vi "ThemalImaging(VDAQ).vi"() -> ()   [LabVIEW 2011]
uses:
  <vilib>/Analysis/1siggen.llb/Riffle Array (I32).vi
  <vilib>/Analysis/NI_AALBase.lvlib
panel:
  in  "选项卡控件":enum32{"前面板", "参数设置"}(tab)
  out "Stim_ID":i32(listbox)=1
  in  "窗口":bool=TRUE
  in  "暂停":bool
  in  "停止":bool
  in  "FramesPerStim":i32=100
  in  "Blk目录":path=path "C:/Documents and Settings/Administrator/桌面/热成像/testblk"
  in  "文件名":string="G4"
  in  "TimeForPrepare(ms)":u32=4000
  in  "InterTrailID":u8
  in  "stim ID":u8[](array[numeric])=[0, 1, 2, 3, 4, 5, 6, 7, 8]
  in  "blk数量":i32=500
  out "错误输出 2":errorcluster
  out "重排的 Stim ID":i32[](array[numeric]) caption="重排的{X}"
  out "重排的 Stim ID Index":i32[](array[numeric]) caption="重排的索引"
  in  "FrameWidth":i32=704
  in  "FrameHeight":i32=576
  in  "Stimuli":i32=5
  out "错误输出":errorcluster
  out "DeInitDSPs":i32
  in  "Brightness":i32(slide) min=0 max=255 scale=0.0..255.0
  in  "Contrast":i32(slide) min=0 max=127 scale=0.0..127.0
  # "开始前一定要改名字"
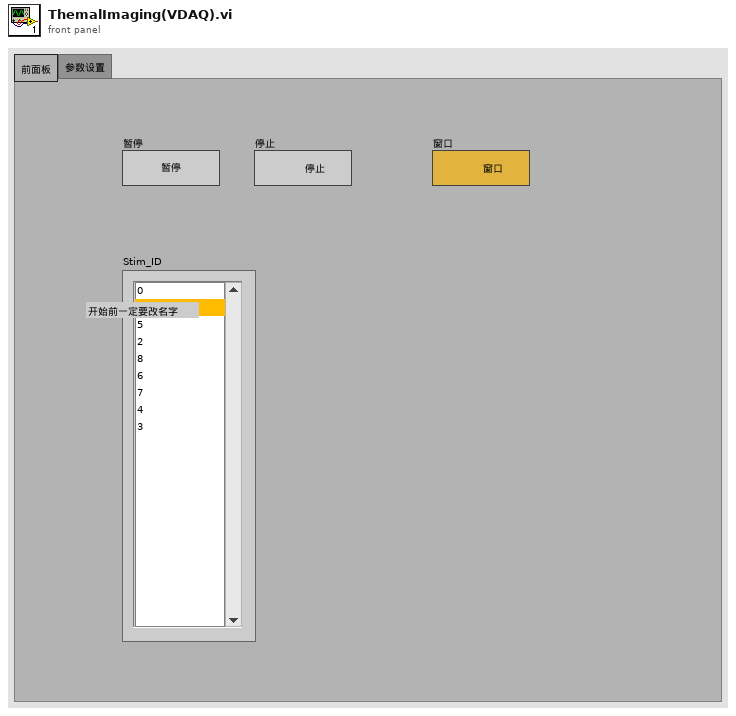
[diagram p1: front panel]
types:
  T1 = typedef "Image Type" = u32
  T2 = typedef "IMAQ Image.ctl" = refnum<image>
  T3 = enum16{"big-endian, network order", "native, host order", "little-endian"}
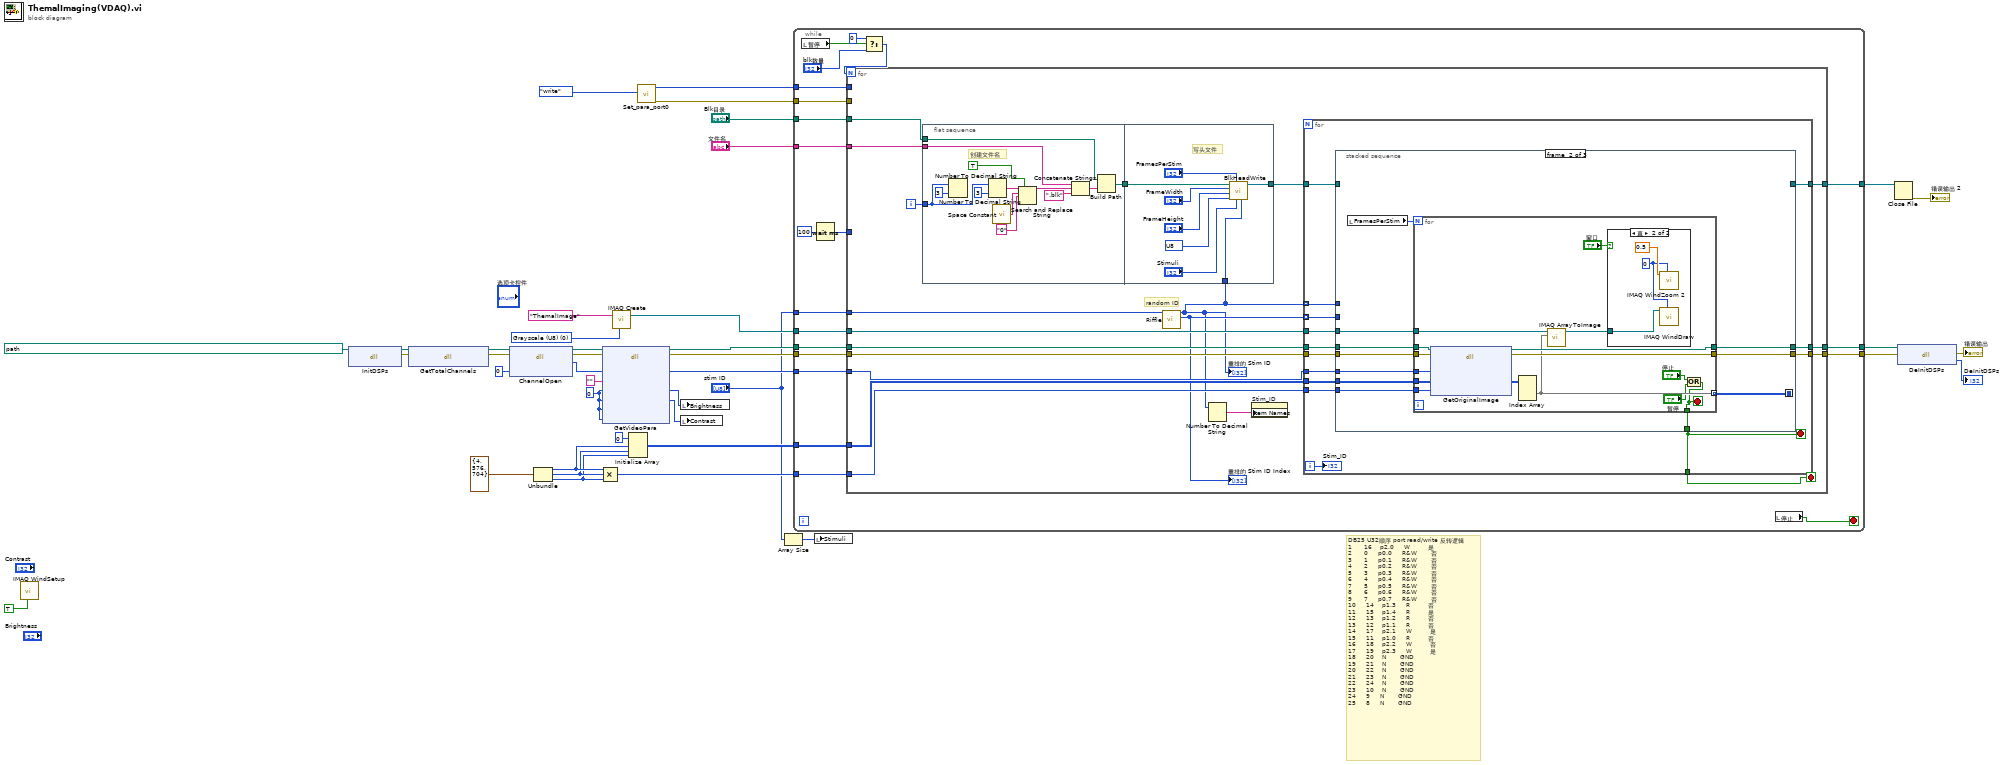
[diagram p0: block diagram]
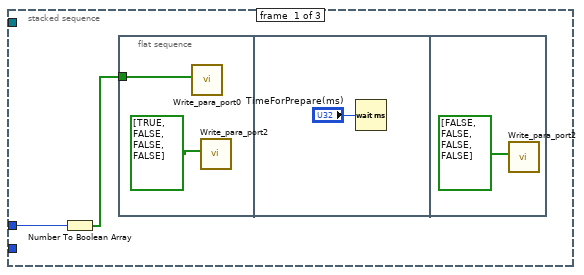
[diagram p2: hidden frame]
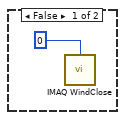
[diagram p3: hidden frame]
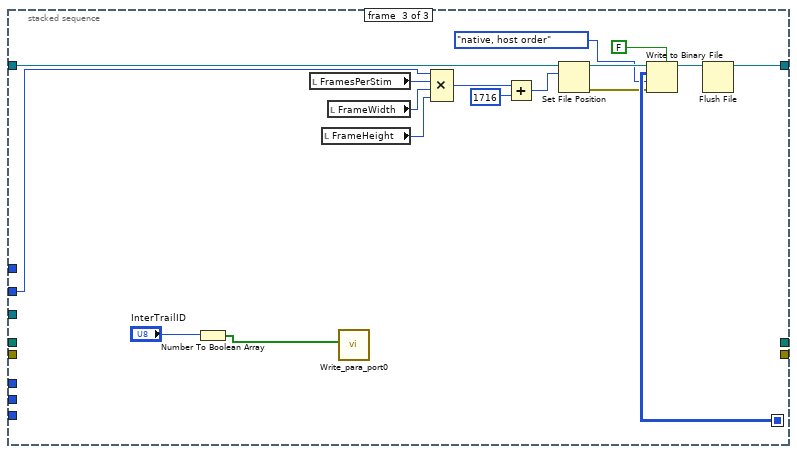
[diagram p4: hidden frame]
diagram:
  w14 = T1 0 items=["Grayscale (U8)", "Grayscale (I16)", "Grayscale (SGL)", "Complex (CSG)", "RGB (U32)", "HSL (U32)", "RGB (U64)", "Grayscale (U16)"] ("Image Type")
  w35 = 0 ("Brightness")
  # "DB25\tU32顺序\tport\tread/write\t反转逻辑\n1\t     16\t   p2.0    \tW\t        是\n2\t     0    \tp0.0\t   \tR&W\t      否\n3\t     1\t\t   p0.1\t   \tR&W      \t否\n4\t\t    2\t   \tp0.2   \t\tR&W      \t否\n5\t\t    3\t\t   p0.3   \t\tR&W\t      否\n6\t\t    4\t   \tp0.4   \t\tR&W      \t否\n7\t\t    5\t   \tp0.5   \t\tR&W      \t否\n8\t\t    6\t   \tp0.6\t   \tR&W      \t否\n9\t    \t7\t   \tp0.7\t   \tR&W\t      否\n10\t    14   \tp1.3   \t\tR        \t否\n11\t   \t15   \tp1.4   \t\tR        \t是\n12\t   \t13   \tp1.2\t   \tR        \t否\n13    \t12   \tp1.1\t   \tR        \t否\n14     17   \tp2.1\t   \tW        \t是\n15    \t11   \tp1.0   \t\tR\t        否\n16    \t18   \tp2.2   \t\tW        \t否\n17    \t19\t   p2.3   \t\tW\t        是\n18    \t20   \tN   \t  \tGND\t\n19    \t21   \tN   \t  \tGND\t\n20\t    22\t   N\t  \t  \tGND\t\n21\t    23\t   N  \t  \t\tGND\t\n22\t    24\t   N  \t  \t\tGND\t\n23    \t10   \tN  \t  \t\tGND\t\n24    \t9\t    N  \t  \t\tGND\t\n25\t    8    \tN  \t  \t\tGND"
  n1 = call "IMAQ WindSetup"("Window is floating? (No)"=TRUE) -> ()  [unwired: 10 in, 1 out]
  n2 = dll-call lib="PTH1labs C\nProgram Files\tHikvision+DS-4000系列板卡SDK and Demo Version 5.1SDKcard sdk\nDs40xxSDK.dll" fn="InitDSPs"(path in=path "C:/Program Files/Hikvision/DS-4000系列板卡SDK and Demo Version 5.1/SDK/card sdk/Ds40xxSDK.dll" ("路径输入")) -> (path out=w39:path, error out=w22:errorcluster)  [unwired: 2 in, 1 out]
  n3 = dll-call lib="PTH1labs C\nProgram Files\tHikvision+DS-4000系列板卡SDK and Demo Version 5.1SDKcard sdk\nDs40xxSDK.dll" fn="GetTotalChannels"(path in=w39, error in=w22) -> (path out=w37:path, error out=w21:errorcluster)  [unwired: 1 in, 1 out]
  n4 = dll-call lib="PTH1labs C\nProgram Files\tHikvision+DS-4000系列板卡SDK and Demo Version 5.1SDKcard sdk\nDs40xxSDK.dll" fn="ChannelOpen"(path in=w37, error in=w21, "ChannelNum"=0) -> (path out=w32:path, error out=w20:errorcluster, "返回类型"=w31:u32)  [unwired: 2 in]
  n5 = Unbundle(cluster{"元素":i32, "元素 2":i32, "元素 3":i32} {"元素"=4, "元素 2"=576, "元素 3"=704}) -> ("元素"=w27:i32, "元素 2"=w26:i32, "元素 3"=w25:i32)
  n6 = dll-call lib="PTH1babs C\nProgram Files\tHikvision+DS-4000系列板卡SDK and Demo Version 5.1Bin\nDs40xxSDK.dll" fn="GetVideoPara"(path in=w32, error in=w20, "hChannelHandle"=w31, "VideoStandard"="", "Brightness"=w35, "Contrast"=w35, "Saturation"=w35, "Hue"=w35) -> (path out=w30:path, error out=w19:errorcluster, "hChannelHandle"=w11:u32, "Brightness"=w33:i32, "Contrast"=w34:i32)  [unwired: 1 in, 4 out]
  n7 = Compound Arithmetic op=MULTIPLY(w27, w26, w25) -> (w23:i32)
  n8 = call "IMAQ Create"("Image Name"="ThemalImage", "Image Type"=w14) -> ("New Image"=w12:T2)  [unwired: 2 in, 2 out]
  n9 = Initialize Array(u8 0 ("元素"), w27, w26, w25) -> (w24:u8[][][])
  n10 = call "Set_para_port0.vi"("R or W"=enum16{"read", "write"}."write") -> ("error out"=w3:errorcluster, "address 2"=w2:i16)  [unwired: 9 in]
  n11 = local write "Brightness"(w33) -> ()
  n12 = local write "Contrast"(w34) -> ()
  n13 = Array Size(array="stim ID") -> (size(s)=w7:i32)
  n14 = while {
    tunnel: w30 -> [w61]
    tunnel: w24 -> [w60]
    tunnel: w23 -> [w59]
    tunnel: w19 -> [w58]
    tunnel: [w57] -> w17
    tunnel: [w56] -> w16
    tunnel: w12 -> [w55]
    tunnel: w11 -> [w54]
    tunnel: [w53] -> w9
    tunnel: "stim ID" -> [w52]
    tunnel: "文件名" -> [w51]
    tunnel: "Blk目录" -> [w50]
    tunnel: w3 -> [w49]
    tunnel: w2 -> [w48]
    stop <- w41 stop-if-true
    n15 = local read "暂停"() -> (w47:bool)
    n16 = Wait (ms)(milliseconds to wait=u32 100 ("等待时间（毫秒）")) -> (millisecond timer value=w42:u32)
    n17 = Select(t=0, s=w47, f="blk数量") -> (s? t:f=w44:i32)
    n18 = for {
      N: w44 -> [_]
      tunnel: w61 -> [w80]
      tunnel: w60 -> [w79]
      tunnel: w59 -> [w78]
      tunnel: w58 -> [w77]
      tunnel: [w76] -> w57
      tunnel: [w75] -> w56
      tunnel: w55 -> [w74]
      tunnel: w54 -> [w73]
      tunnel: [w72] -> w53
      tunnel: w52 -> [w71]
      tunnel: w51 -> [w69]
      tunnel: w50 -> [w68]
      tunnel: w49 -> [_]
      tunnel: w48 -> [_]
      tunnel: w42 -> [_]
      i -> [w70]
      stop <- w62 stop-if-true
      # "random ID"
      n19 = flat-sequence {
        tunnel: w70 -> [w87]
        tunnel: w69 -> [w86]
        tunnel: w68 -> [w82]
        tunnel: [w81] -> w66
        tunnel: w66 -> [w96]
        tunnel: [w95] -> w65
        tunnel: w64 -> [w94]
        frame #0 {
          # "创建文件名"
          n20 = Number To Decimal String(number=w87, width (-)=i16 3 ("宽度(-)")) -> ()  [unwired: 1 out]
          n21 = Number To Decimal String(number=w87, width (-)=i16 3 ("宽度(-)")) -> (decimal integer string=w89:string)
          n22 = call <vilib>:"Space Constant.vi"() -> ("String"=w90:string)
          n23 = Search and Replace String(replace all?=TRUE ("替换全部？(F)"), input string=w89, search string=w90, replace string="0" ("替换字符串(\"\")")) -> (result string=w85:string)  [unwired: 4 in, 3 out]
          n24 = Concatenate Strings(w86, w85, ".blk" ("字符串")) -> (w83:string)
          n25 = Build Path(base path=w82, name or relative path=w83) -> (appended path=w81:path)
        }
        frame #1 {
          w99 = u16 11 items=["U8"=11, "I16"=12, "U32"=13, "SGL"=14] ("datatype")
          # "写头文件"
          n26 = call "BlkHeadWrite.vi"("SequenceOfID"=w94, "Stimuli"="Stimuli", "FramesPerStim"="FramesPerStim", "datatype"=w99, "FrameHeight"="FrameHeight", "FrameWidth"="FrameWidth", "BlkFilePath"=w96) -> ("引用句柄输出"=w95:refnum<file>)  [unwired: 4 in]
        }
      }
      n27 = call-poly <vilib>:"Riffle.vi"("X"=w71) -> ("Riffled Index"=w67:i32[], "Riffled {X}"=w64:i32[])  [unwired: 8 in, 1 out]
      "重排的 Stim ID Index" <- w67
      "重排的 Stim ID" <- w64
      n28 = Number To Decimal String(number=w64) -> (decimal integer string=w63:string[])  [unwired: 1 in]
      n29 = property on="Stim_ID" class="LstBox (严格)"("Item Names"=w63) -> ()  [unwired: 2 in, 2 out]
      n30 = for {
        tunnel: w80 -> [w115]
        tunnel: w79 -> [w114]
        tunnel: w78 -> [w113]
        tunnel: w77 -> [w112]
        tunnel: [w106] -> w76
        tunnel: [w105] -> w75
        tunnel: w74 -> [w111]
        tunnel: w73 -> [w110]
        tunnel: w65 -> [w109]
        tunnel: [w107] -> w72
        tunnel: w67 -> [w108] mode=indexing
        tunnel: w64 -> [w104] mode=indexing
        tunnel: [w103] -> w62
        i -> [w102]
        stop <- w103 stop-if-true
        n31 = stacked-sequence {
          seq-local: [_ w126 _] -> [_ _ w168]
          tunnel: w115 -> [_ w132 _]
          tunnel: w114 -> [_ w131 _]
          tunnel: w113 -> [_ w130 _]
          tunnel: w112 -> [_ w129 _]
          tunnel: w111 -> [_ w128 _]
          tunnel: w110 -> [_ w127 _]
          tunnel: w109 -> [_ _ w167]
          tunnel: w108 -> [_ _ w166]
          tunnel: [_ _ w152] -> w107
          tunnel: [_ w124 _] -> w106
          tunnel: [_ w123 _] -> w105
          tunnel: w104 -> [w117 _ _]
          tunnel: [_ w122 _] -> w103
          frame #0 {
            n32 = Number To Boolean Array(number=w117) -> (Boolean array=w116:bool[])
            n33 = flat-sequence {
              tunnel: w116 -> [w119]
              frame #0 {
                n34 = call "Write_para_port0.vi"("port0（8元素）"=w119) -> ()  [unwired: 10 in, 1 out]
                n35 = call "Write_para_port2.vi"("port2（4元素）"=bool[] [TRUE, FALSE, FALSE, FALSE] ("port2")) -> ()  [unwired: 10 in, 1 out]
              }
              frame #1 {
                n36 = Wait (ms)(milliseconds to wait="TimeForPrepare(ms)") -> ()  [unwired: 1 out]
              }
              frame #2 {
                n37 = call "Write_para_port2.vi"("port2（4元素）"=bool[] [FALSE, FALSE, FALSE, FALSE] ("port2")) -> ()  [unwired: 10 in, 1 out]
              }
            }
          }
          frame #1 {
            n38 = local read "FramesPerStim"() -> (w125:i32)
            n39 = for {
              N: w125 -> [_]
              tunnel: w132 -> [w147]
              tunnel: w131 -> [w146]
              tunnel: w130 -> [w145]
              tunnel: w127 -> [w144]
              tunnel: w129 -> [w143]
              tunnel: [w142] -> w124
              tunnel: [w141] -> w123
              tunnel: w128 -> [w139]
              tunnel: [w136] -> w126 mode=indexing
              tunnel: [w133] -> w122
              stop <- w133 stop-if-true
              n40 = dll-call lib="PTH1labs C\nProgram Files\tHikvision+DS-4000系列板卡SDK and Demo Version 5.1SDKcard sdk\nDs40xxSDK.dll" fn="GetOriginalImage"(path in=w147, error in=w143, "hChannelHandle"=w144, "ImageBuf"=w146, "Size"=w145) -> (path out=w142:path, error out=w141:errorcluster, "ImageBuf"=w140:u8[][][])  [unwired: 2 in, 2 out]
              n41 = Index Array(array=w140) -> (element=w136:u8[][])  [unwired: 3 in]
              n42 = call "IMAQ ArrayToImage"("Image Pixels (U8)"=w136, "Image"=w139) -> ("Image Out"=w138:T2)  [unwired: 4 in, 5 out]
              n43 = case shown="真" "窗口" {
                tunnel: w138 -> [_ w151]
                frame False {
                  n44 = call "IMAQ WindClose"("Window Number (0...15)"=0) -> ()  [unwired: 5 in, 1 out]
                }
                frame True {
                  w149 = 0 ("Window Number (0...15)")
                  n45 = call "IMAQ WindZoom 2"("Window Number (0...15)"=w149, "Zoom Factor"=sgl 0.5) -> ()  [unwired: 6 in, 4 out]
                  n46 = call "IMAQ WindDraw"("Window Number (0...15)"=w149, "Image"=w151) -> ()  [unwired: 8 in, 2 out]
                }
              }
              n47 = Or(x="停止", y="暂停") -> (x .or. y?=w133:bool)
            }
          }
          frame #2 {
            n48 = Number To Boolean Array(number="InterTrailID") -> (Boolean array=w154:bool[])
            n49 = local read "FramesPerStim"() -> (w158:i32)
            n50 = local read "FrameHeight"() -> (w156:i32)
            n51 = local read "FrameWidth"() -> (w157:i32)
            n52 = call "Write_para_port0.vi"("port0（8元素）"=w154) -> ()  [unwired: 10 in, 1 out]
            n53 = Compound Arithmetic op=MULTIPLY(w166, w158, w157, w156) -> (w161:i32)
            n54 = Add(x=w161, y=i64 1716 ("偏移量（字节）（0）")) -> (x+y=w159:i64)
            n55 = Set File Position(offset (in bytes) (0)=w159, refnum=w167) -> (refnum out=w164:refnum<file>, error out=w162:errorcluster)  [unwired: 2 in]
            n56 = Write to Binary File(file (use dialog)=w164, data=w168, error in=w162, 5:FALSE ("预置数组或字符串大小？(T)"), 9:T3."native, host order" ("字节顺序(0:big-endian, network order)")) -> (refnum out=w153:refnum<file>)  [unwired: 1 in, 2 out]
            n57 = Flush File(refnum=w153) -> (refnum out=w152:refnum<file>)  [unwired: 1 in, 1 out]
          }
        }
        "Stim_ID" <- w102
      }
    }
    n58 = local read "停止"() -> (w41:bool)
  }
  n59 = local write "Stimuli"(w7) -> ()
  n60 = Close File(refnum=w9) -> (error out=→"错误输出 2":errorcluster)  [unwired: 1 in, 1 out]
  n61 = dll-call lib="PTH1labs C\nProgram Files\tHikvision+DS-4000系列板卡SDK and Demo Version 5.1SDKcard sdk\nDs40xxSDK.dll" fn="DeInitDSPs"(path in=w17, error in=w16) -> (error out=→"错误输出":errorcluster, "返回类型"=→"DeInitDSPs":i32)  [unwired: 1 in, 1 out]
